vi "Move arm to position.vi"(7 "Description":string, 8 "Command Info In":T2, 11 "Arm Position":T1=enum."Hatch - Ground") -> (0 "Command Info Out":T2)   [LabVIEW 2018]
doc: "This template is useful for immediate subsystem actions that do not need deadband filtering\n\nBe sure to right-click and select New from Template and save with a new command name."
uses:
  <vilib>/Rock Robotics/WPI/Framework/Command Status Info.ctl
  <vilib>/Rock Robotics/WPI/Framework/Completion Status.ctl
  <vilib>/Rock Robotics/WPI/Framework/Completion Notifier.ctl
  Arm Positions.ctl
  Implementation/Arm Setpoints.ctl
  Implementation/Arm Operations.ctl
  Implementation/Arm Published Globals.vi
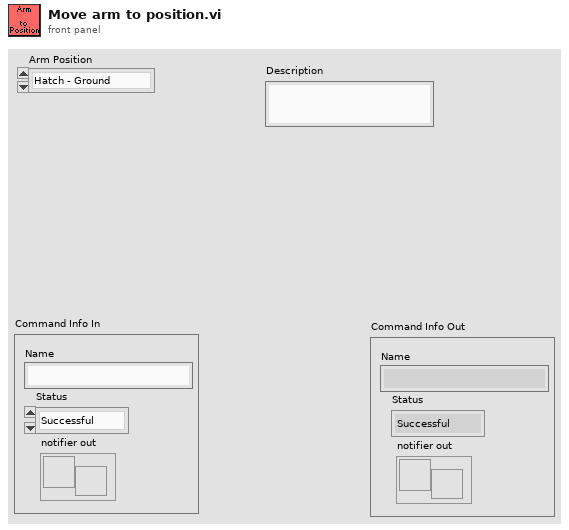
[diagram p1: front panel]
types:
  T1 = typedef "Arm Positions.ctl" = enum16{"Home Position", "Hatch - Ground", "Hatch - Low", "Hatch - Middle", "Hatch - High", "Cargo - Low", "Cargo - Middle", "Cargo - High", "Cargo - Loading Station", "Cargo - Ground", "Turret - Left", "Turret - Front", "Turret - Right", "Turret - Back", "Climbing - Forward"}
  T2 = typedef "Command Status Info.ctl" = cluster{"Name":string, "Status":T3, "notifier out":T4}
  T3 = typedef "Completion Status.ctl" = enum16{"Successful", "Aborted", "Incomplete"}
  T4 = typedef "Completion Notifier.ctl" = refnum<notifier>
  T5 = typedef "Arm Setpoints.ctl" = cluster{"Operation":T6, "Turret Setpoint":dbl, "Shoulder Setpoint":dbl, "Elbow Setpoint":dbl, "Wrist Setpoint":dbl}
  T6 = typedef "Arm Operations.ctl" = enum16{"Reserve", "Read Current", "Immediate", "Move arm to position"}
  T7 = cluster{"Current Command":T5, "Command Timing":cluster{"Start Time (ms)":u32, "Iterations":i32}, "Command Arguments":cluster{"Command Info":T2, "Description":string, "Default Command":T5, "queue out":refnum<queue>, "Subsystem Name":string}}
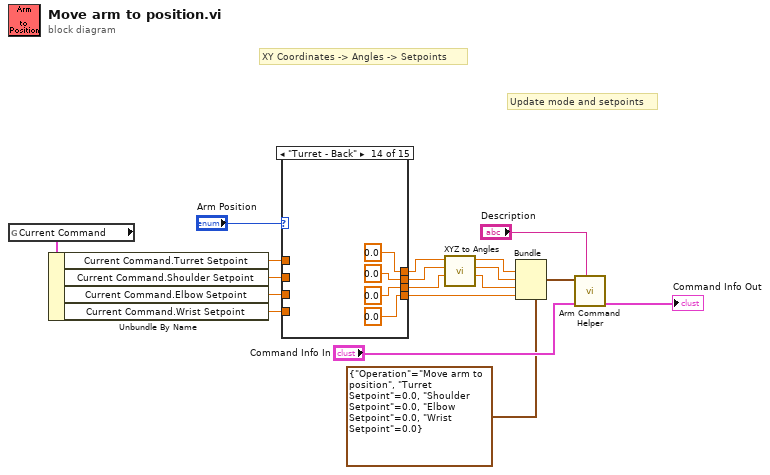
[diagram p0: block diagram]
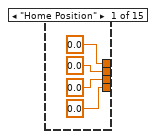
[diagram p2: hidden frame]
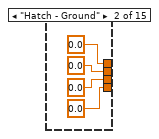
[diagram p3: hidden frame]
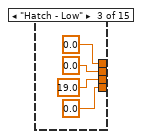
[diagram p4: hidden frame]
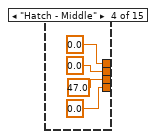
[diagram p5: hidden frame]
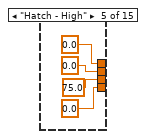
[diagram p6: hidden frame]
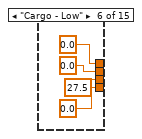
[diagram p7: hidden frame]
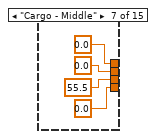
[diagram p8: hidden frame]
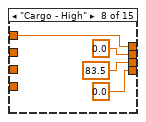
[diagram p9: hidden frame]
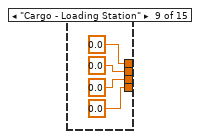
[diagram p10: hidden frame]
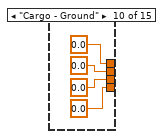
[diagram p11: hidden frame]
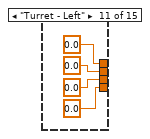
[diagram p12: hidden frame]
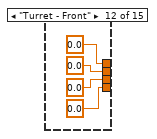
[diagram p13: hidden frame]
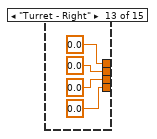
[diagram p14: hidden frame]
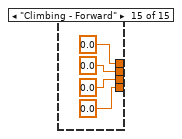
[diagram p15: hidden frame]
diagram:
  # "XY Coordinates -> Angles -> Setpoints"
  # "Update mode and setpoints"
  n1 = global read "Arm Published Globals.vi" "Current Command"() -> (w5:T7)
  n2 = Unbundle By Name(w5) -> ("Current Command.Turret Setpoint"=w4:dbl, "Current Command.Shoulder Setpoint"=w3:dbl, "Current Command.Elbow Setpoint"=w2:dbl, "Current Command.Wrist Setpoint"=w1:dbl)
  n3 = case shown="\"Turret - Back\"" "Arm Position" {
    tunnel: [0.0 0.0 0.0 0.0 0.0 0.0 0.0 w47 0.0 0.0 0.0 0.0 0.0 0.0 0.0] -> w11
    tunnel: [0.0 0.0 0.0 0.0 0.0 0.0 0.0 0.0 0.0 0.0 0.0 0.0 0.0 0.0 0.0] -> w9
    tunnel: [0.0 0.0 0.0 0.0 0.0 0.0 0.0 0.0 0.0 0.0 0.0 0.0 0.0 0.0 0.0] -> w12
    tunnel: [0.0 0.0 19.0 47.0 75.0 27.5 55.5 83.5 0.0 0.0 0.0 0.0 0.0 0.0 0.0] -> w7
    tunnel: w4 -> [_ _ _ _ _ _ _ w47 _ _ _ _ _ _ _]
    tunnel: w3 -> [_ _ _ _ _ _ _ _ _ _ _ _ _ _ _]
    tunnel: w2 -> [_ _ _ _ _ _ _ _ _ _ _ _ _ _ _]
    tunnel: w1 -> [_ _ _ _ _ _ _ _ _ _ _ _ _ _ _]
    frame "Home Position" {
    }
    frame "Hatch - Ground" {
    }
    frame "Hatch - Low" {
    }
    frame "Hatch - Middle" {
    }
    frame "Hatch - High" {
    }
    frame "Cargo - Low" {
    }
    frame "Cargo - Middle" {
    }
    frame "Cargo - High" {
    }
    frame "Cargo - Loading Station" {
    }
    frame "Cargo - Ground" {
    }
    frame "Turret - Left" {
    }
    frame "Turret - Front" {
    }
    frame "Turret - Right" {
    }
    frame "Turret - Back" {
    }
    frame "Climbing - Forward" {
    }
  }
  n4 = call "XYZ to Angles.vi"("Z Target Position"=w7, "Y Target Position"=w9, "X Target Position"=w11) -> ("Elbow Angle"=w6:dbl, "Shoulder Angle"=w8:dbl, "Turret Angle"=w10:dbl)  [unwired: 6 in]
  n5 = Bundle(cluster=T5 {"Operation"=enum."Move arm to position", "Turret Setpoint"=0.0, "Shoulder Setpoint"=0.0, "Elbow Setpoint"=0.0, "Wrist Setpoint"=0.0} ("SubSystem Data"), "Turret Setpoint"=w10, "Shoulder Setpoint"=w8, "Elbow Setpoint"=w6, "Wrist Setpoint"=w12) -> (w14:T5)  [unwired: 1 in]
  n6 = call "Arm Command Helper.vi"("Description"="Description", "Command Info In"="Command Info In", "SubSystem Data"=w14) -> ("Command Info Out"=→"Command Info Out":T2)  [unwired: 6 in, 2 out]
